vi "Configure Relay Name Lookup.vi"(8 "error in (no error)":errorcluster, 9 "K2 ChannelName":string, 10 "K1 ChannelName":string, 11 "TCP 380 in":refnum<class "TCP 380.lvclass">) -> (0 "error out":errorcluster, 3 "TCP 380 out":refnum<class "TCP 380.lvclass">)   [LabVIEW 2021, in "TCP 380.lvclass"]
uses:
  TCP 380.lvclass
  TCP 380.lvclass/TCP 380.ctl
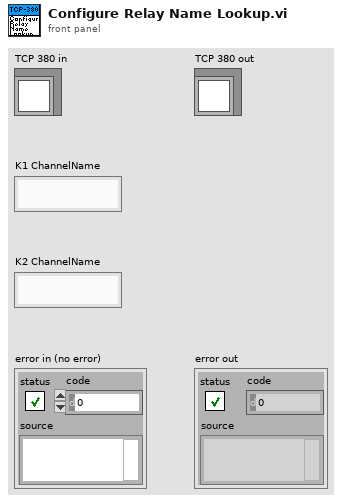
[diagram p1: front panel]
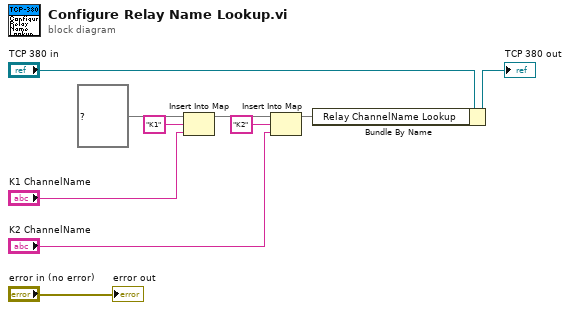
[diagram p0: block diagram]
diagram:
  n1 = Insert Into Map(map in=map{string, string} {} ("Relay ChannelName Lookup"), key="K1", value="K1 ChannelName") -> (map out=w7:map{string, string})  [unwired: 2 out]
  n2 = Insert Into Map(map in=w7, key="K2", value="K2 ChannelName") -> (map out=w5:map{string, string})  [unwired: 2 out]
  n3 = Bundle By Name(cluster="TCP 380 in", "Relay ChannelName Lookup"=w5) -> (→"TCP 380 out":refnum<class "TCP 380.lvclass">)
  "error out" <- "error in (no error)"
